vi "Matr_col.vi"(2 "Coloana":u8, 3 "Date":u8, 4 "Adresa":u32) -> (0 "Numeric":u8, 1 "Numeric 2":u8)   [LabVIEW 2009]
uses:
  <vilib>/Platform/portaccess.llb/Out Port8.vi
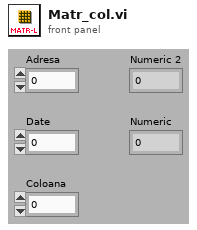
[diagram p1: front panel]
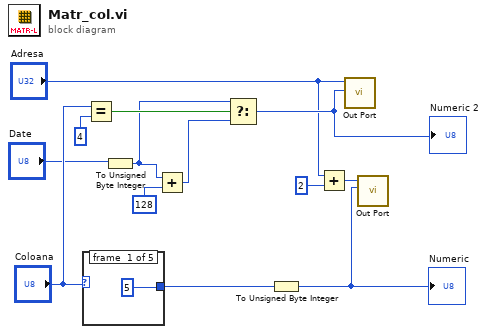
[diagram p0: block diagram]
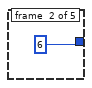
[diagram p2: hidden frame]
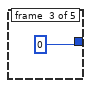
[diagram p3: hidden frame]
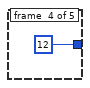
[diagram p4: hidden frame]
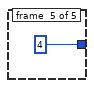
[diagram p5: hidden frame]
diagram:
  n1 = case shown="0, Default" "Coloana" {
    tunnel: [5 6 0 12 4] -> w1
    frame #0 {
    }
    frame #1 {
    }
    frame #2 {
    }
    frame #3 {
    }
    frame #4 {
    }
  }
  n2 = Equal?(x="Coloana", y=u8 4) -> (x = y?=w8:bool)
  n3 = To Unsigned Byte Integer(number="Date") -> (unsigned 8bit integer=w5:u8)
  n4 = Add(x=w5, y=u8 128) -> (x+y=w6:u8)
  n5 = Select(t=w5, s=w8, f=w6) -> (s? t:f=w12:u8)
  "Numeric 2" <- w12
  n6 = To Unsigned Byte Integer(number=w1) -> (unsigned 8bit integer=w13:u8)
  "Numeric" <- w13
  n7 = Add(x="Adresa", y=u8 2) -> (x+y=w3:u32)
  n8 = call-poly <vilib>:"Out Port.vi"("write value"=w12, "address"="Adresa") -> ()  [unwired: 7 in, 1 out]
  n9 = call-poly <vilib>:"Out Port.vi"("write value"=w13, "address"=w3) -> ()  [unwired: 7 in, 1 out]
